vi "4.2 Float with Unit CSM API String to Float.vi"() -> ()   [LabVIEW 2017]
uses:
  addons/API-String-Arugments-Support/API String Arguments Support.lvlib
panel:
  out "Example List":T1(array[cluster])=[{"CSM API String"="1.24A", "Float"=1.24, "Unit String"="A"}, {"CSM API String"="1.2KHz", "Float"=1200.0, "Unit String"="Hz"}, {"CSM API String"="1.2kHz", "Float"=1200.0, "Unit String"="Hz"}, {"CSM API String"="1.2 kHz", "Float"=1.2, "Unit String"="kHz"}, {"CSM API String"="243Ω", "Float"=243.0, "Unit String"="Ω"}, {"CSM API String"="12 mV", "Float"=12.0, "Unit String"="mV"}, {"CSM API String"="12mV", "Float"=0.012, "Unit String"="V"}, {"CSM API String"="1.23456435E+5A", "Float"=123456.43500000001, "Unit String"="A"}, {"CSM API String"="1.23456435E+5mA", "Float"=123456.43500000001, "Unit String"="mA"}, {"CSM API String"="1.23456435E+5 mA", "Float"=123456.43500000001, "Unit String"="mA"}]
  # "#CSM-Example Overview\n\n本范例演示API String中包含单位的浮点数转换为浮点数的示例。"
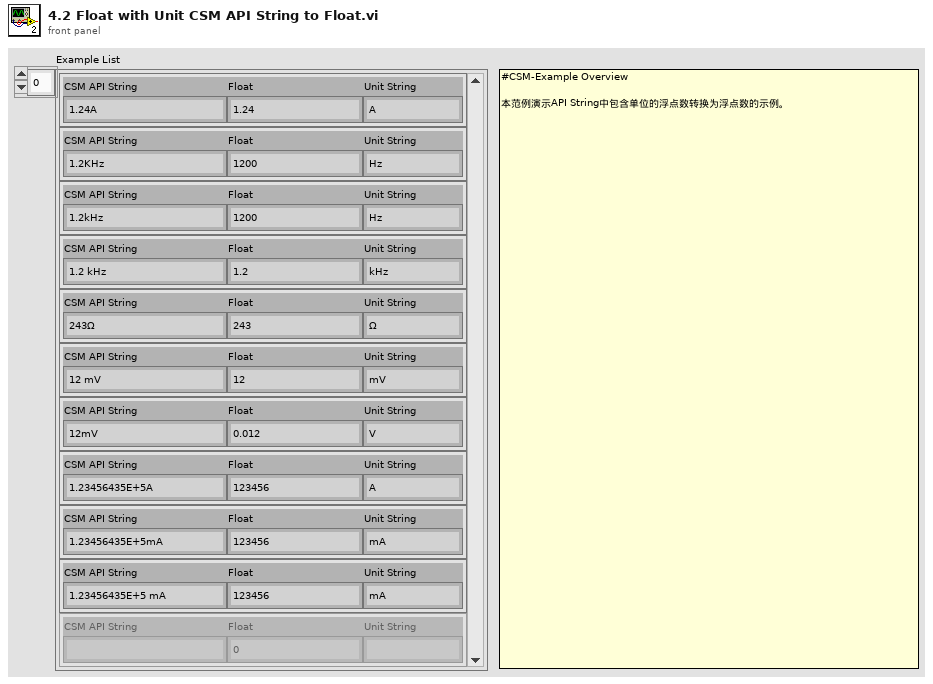
[diagram p1: front panel]
types:
  T1 = cluster{"CSM API String":string, "Float":dbl, "Unit String":string}[]
  T2 = cluster{"String":string, "Float":dbl, "Unit String":string}
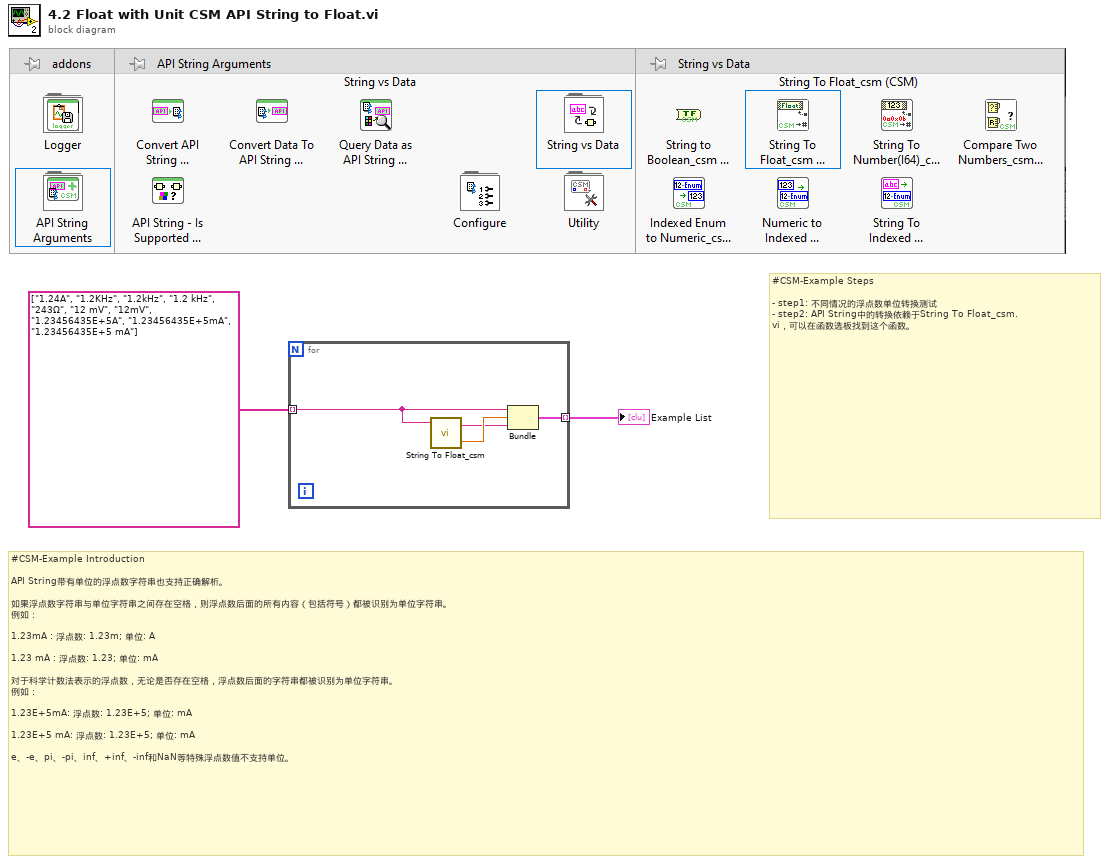
[diagram p0: block diagram]
diagram:
  # "#CSM-Example Steps\n\n- step1: 不同情况的浮点数单位转换测试\n- step2: API String中的转换依赖于String To Float_csm.vi，可以在函数选板找到这个函数。"
  # "#CSM-Example Introduction\n\nAPI String带有单位的浮点数字符串也支持正确解析。\n\n如果浮点数字符串与单位字符串之间存在空格，则浮点数后面的所有内容（包括符号）都被识别为单位字符串。\n例如：\n\n1.23mA : 浮点数: 1.23m; 单位: A \n\n1.23 mA : 浮点数: 1.23; 单位: mA\n\n对于科学计数法表示的浮点数，无论是否存在空格，浮点数后面的字符串都被识别为单位字符串。\n例如：\n\n1.23E+5mA: 浮点数: 1.23E+5; 单位: mA \n\n1.23E+5 mA: 浮点数: 1.23E+5; 单位: mA\n\ne、-e、pi、-pi、inf、+inf、-inf和NaN等特殊浮点数值不支持单位。"
  n1 = for {
    tunnel: string[] ["1.24A", "1.2KHz", "1.2kHz", "1.2 kHz", "243Ω", "12 mV", "12mV", "1.23456435E+5A", "1.23456435E+5mA", "1.23456435E+5 mA"] ("String") -> [w5] mode=indexing
    tunnel: [w6] -> w1 mode=indexing
    n2 = call "String To Float_csm.vi"("String"=w5) -> ("Float"=w4:dbl, "Unit String"=w3:string)  [unwired: 3 in]
    n3 = Bundle("String"=w5, "Float"=w4, "Unit String"=w3) -> (w6:T2)  [unwired: 1 in]
  }
  "Example List" <- w1
